vi "Interactive LED bar graph.vi"() -> ()   [LabVIEW 2010]
doc: "This example shows how to make a bar graph by controlling Red Pitaya on board LEDs.\nThe number of LEDs that will be turned ON, corresponds to the value of variable p\nthat can be set by LabVIEW slider bar."
uses:
  RedPitaya.lvlib
panel:
  in  "stop":bool
  in  "Value":i32(slide) scale=0.0..100.0
  in  "IP address":string="192.168.4.129"
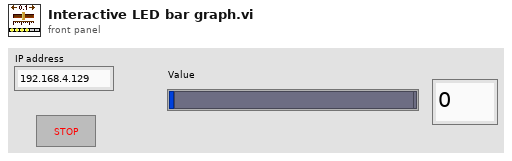
[diagram p1: front panel]
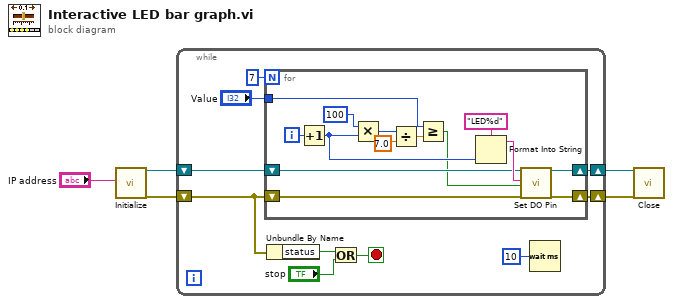
[diagram p0: block diagram]
diagram:
  n1 = call "Initialize.vi"("IP address"="IP address") -> ("RedPitaya TCP Connection"=w2:refnum<k5>, "error out"=w1:errorcluster)  [unwired: 17 in]
  n2 = while {
    shift-right: [w15] -> w4
    shift-left: w2 -> [w13]
    shift-right: [w14] -> w3
    shift-left: w1 -> [w9]
    stop <- w6 stop-if-true
    n3 = for {
      N: 7 -> [_]
      tunnel: "Value" -> [w25]
      shift-right: [w19] -> w15
      shift-left: w13 -> [w20]
      shift-right: [w18] -> w14
      shift-left: w9 -> [w21]
      i -> [w23]
      n4 = Increment(x=w23) -> (x+1=w17:i32)
      n5 = Multiply(x=100, y=w17) -> (x*y=w27:i32)
      n6 = Divide(x=w27, y=7.0) -> (x/y=w29:dbl)
      n7 = Greater Or Equal?(x=w25, y=w29) -> (x >= y?=w16:bool)
      n8 = Format Into String(format string="LED%d", w17) -> (resulting string=w22:string)  [unwired: 2 in, 1 out]
      n9 = call "Set DO Pin.vi"("RedPitaya connection in"=w20, "Pin #"=w22, "State"=w16, "error in"=w21) -> ("RedPitaya connection out"=w19:refnum<k5>, "error out"=w18:errorcluster)  [unwired: 14 in]
    }
    n10 = Unbundle By Name(w9) -> ("status"=w8:bool)
    n11 = Or(x=w8, y="stop") -> (x .or. y?=w6:bool)
    n12 = Wait (ms)(milliseconds to wait=u32 10) -> ()  [unwired: 1 out]
  }
  n13 = call "Close.vi"("connection ID"=w4, "error in"=w3) -> ()  [unwired: 17 in, 1 out]
